vi "TX-ADAR-DETECT.vi"(0 "COMPORT":refnum<visa-resource-name>="COM4", 11 "error in (no error)":errorcluster, 12 "Ant_Sel":i32=1, 13 "Open/Close Serial":bool) -> (3 "string":string="wr txm 0x4A 0x76;wr txm 0x49 0x72", 4 "comport":refnum<visa-resource-name>="COM4", 8 "adc read":dbl=86.0, 15 "error out":errorcluster)   [LabVIEW 2018]
panel:
  out "number":i32=86
  out "after substring":string="56\r\n>\r\n"
  out "All Success":bool=TRUE
  out "output 2":string="\rwr txm 0x4A 0x76\r\n>\rwr txm 0x49 0x72\r\n>\r\rwr txm 0x4A 0x76\r\n>\rwr txm 0x49 0x72\r\n>\rrd txm 0x4B\r\n0x04B: 0x56\r\n>"
  out "Success":bool[](array[boolean])=[TRUE, TRUE, TRUE, TRUE, TRUE, TRUE]
  # "0 for temperature, 13 for Testport"
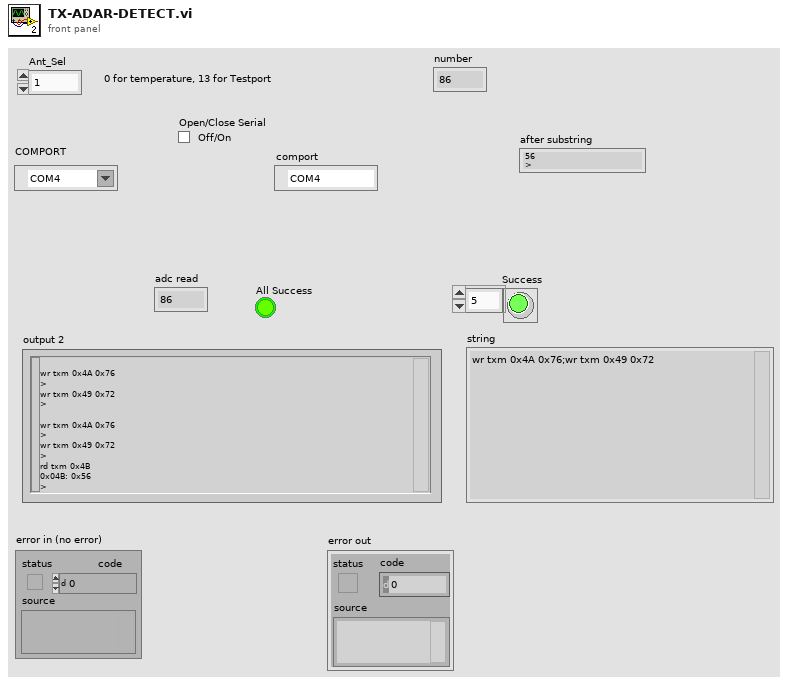
[diagram p1: front panel]
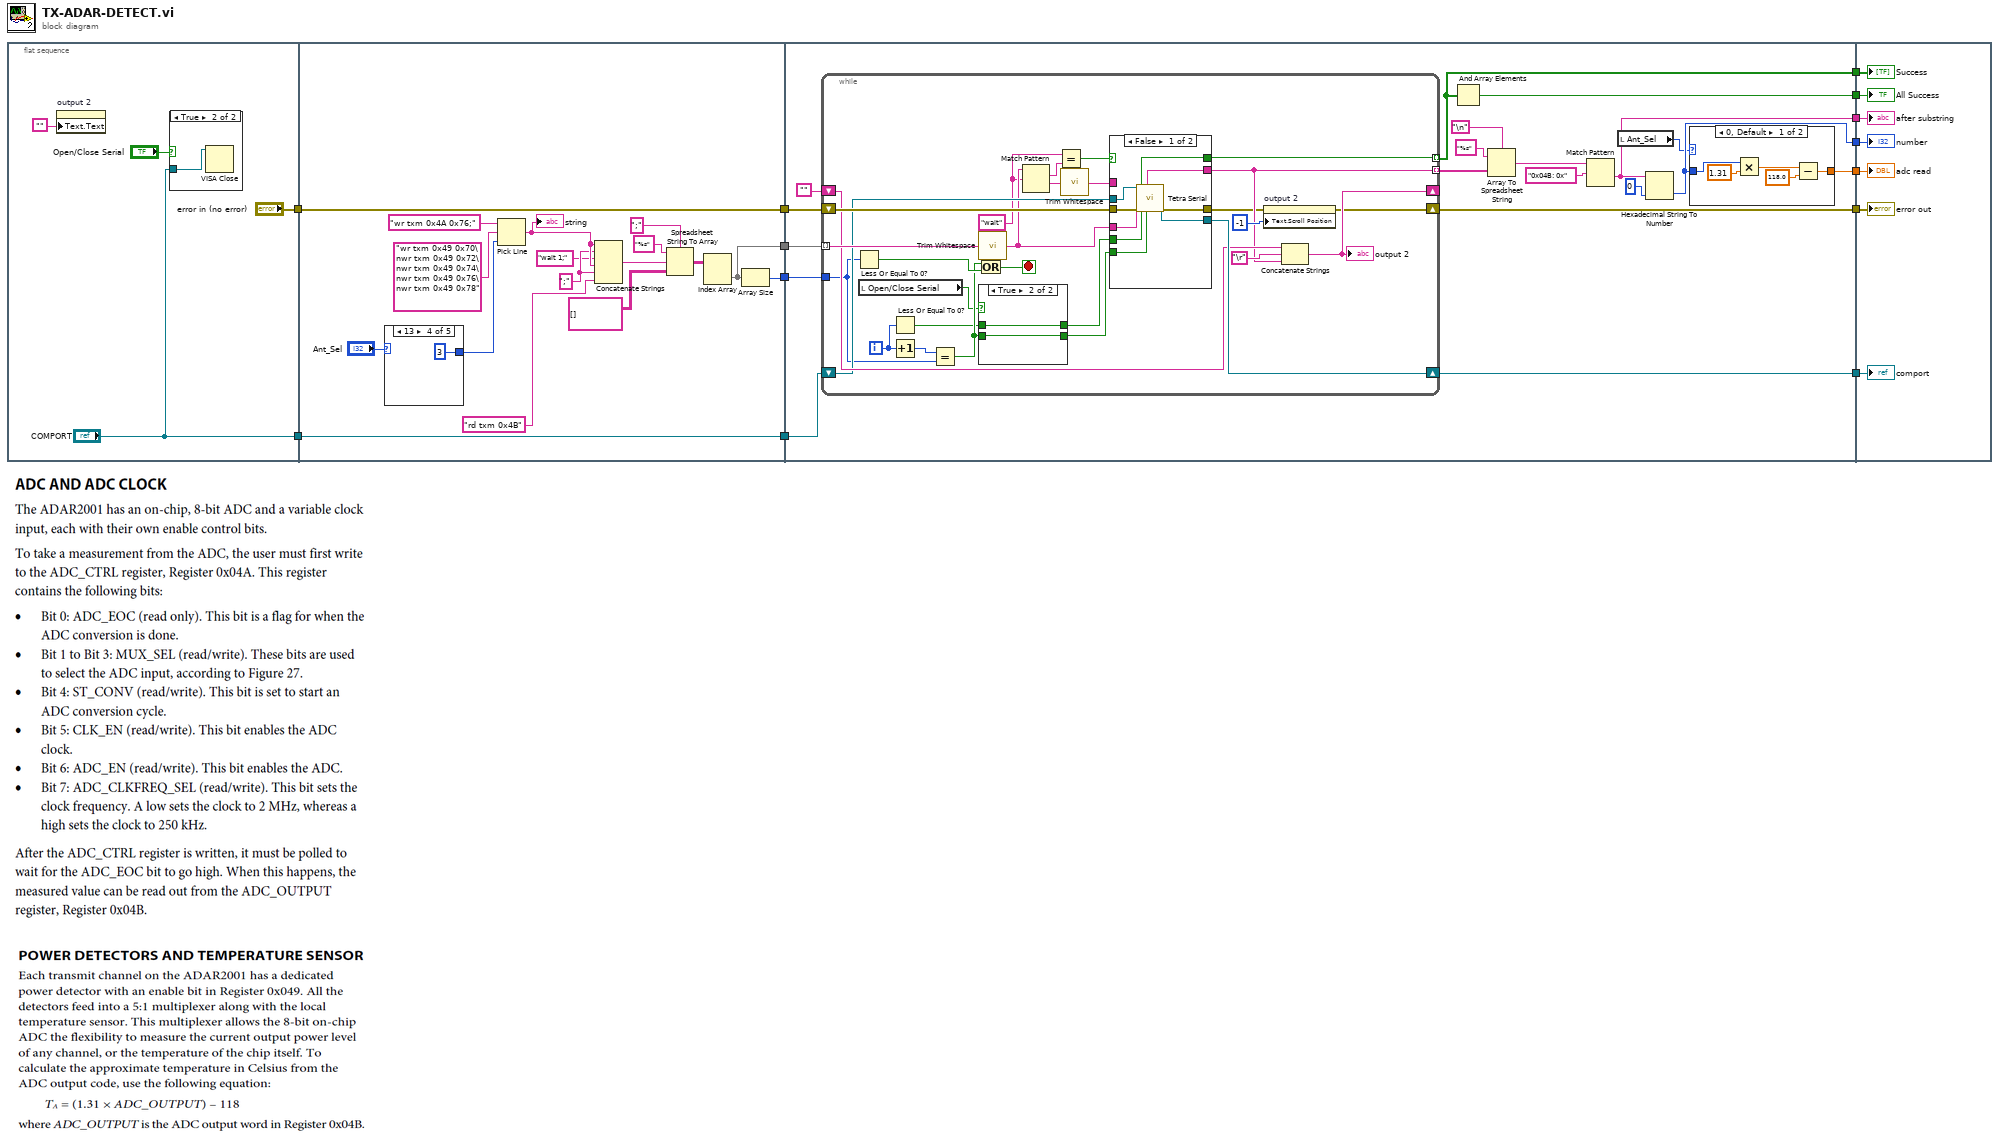
[diagram p0: block diagram]
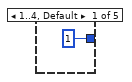
[diagram p3: hidden frame]
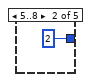
[diagram p4: hidden frame]
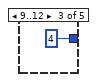
[diagram p5: hidden frame]
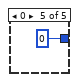
[diagram p6: hidden frame]
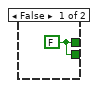
[diagram p8: hidden frame]
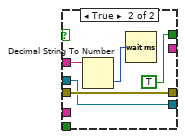
[diagram p9: hidden frame]
diagram:
  n1 = flat-sequence {
    tunnel: ["COMPORT"] -> w2
    tunnel: ["error in (no error)"] -> w1
    tunnel: [w19] -> w6
    tunnel: [w21] -> w5
    tunnel: [w22] -> w4
    tunnel: [w20] -> w3
    tunnel: w2 -> [w20]
    tunnel: w1 -> [w19]
    tunnel: [w59] -> w13
    tunnel: [w57] -> w12
    tunnel: [w52] -> w11
    tunnel: [w51] -> w10
    tunnel: [w46] -> w9
    tunnel: [w44] -> w8
    tunnel: [w43] -> w7
    tunnel: w6 -> [w58]
    tunnel: w5 -> [w56]
    tunnel: w4 -> [w49]
    tunnel: w3 -> [w41]
    tunnel: w13 -> [w111]
    tunnel: w12 -> [w112]
    tunnel: w11 -> [w113]
    tunnel: w10 -> [w114]
    tunnel: w9 -> [w115]
    tunnel: w8 -> [w117]
    tunnel: w7 -> [w116]
    frame #0 {
      n2 = property on="output 2" class="Str"("Text.Text"="") -> ()  [unwired: 2 in, 2 out]
      n3 = case shown="True" "Open/Close Serial" {
        tunnel: "COMPORT" -> [_ w18]
        frame False {
        }
        frame True {
          n4 = VISA Close(VISA resource name=w18) -> ()  [unwired: 1 in, 1 out]
        }
      }
    }
    frame #1 {
      w28 = ";" ("string")
      n5 = case shown="13" "Ant_Sel" {
        tunnel: [1 2 4 3 0] -> w34
        frame 1..4, Default {
        }
        frame 5..8 {
        }
        frame 9..12 {
        }
        frame 13 {
        }
        frame 0 {
        }
      }
      n6 = Pick Line(string ("")="wr txm 0x4A 0x76;" ("Command ( ; seperation)"), multi-line string="wr txm 0x49 0x70\nwr txm 0x49 0x72\nwr txm 0x49 0x74\nwr txm 0x49 0x76\nwr txm 0x49 0x78", line index=w34) -> (output string=w35:string)
      "string" <- w35
      n7 = Concatenate Strings(w35, w28, "wait 1;" ("string"), w35, w28, "rd txm 0x4B" ("string")) -> (w32:string)
      n8 = Spreadsheet String To Array(delimiter (Tab)=";", format string="%s", spreadsheet string=w32, array type (2D Dbl)=string[][] []) -> (array=w31:string[][])
      n9 = Index Array(array=w31) -> (element=w21:string[])  [unwired: 2 in]
      n10 = Array Size(array=w21) -> (size(s)=w22:i32)
    }
    frame #2 {
      n11 = while {
        shift-right: [w71] -> w59
        shift-left: w58 -> [w93]
        shift-right: [w92] -> w57
        shift-left: w41 -> [w82]
        tunnel: [w87] -> w50 mode=indexing
        tunnel: w56 -> [w91] mode=indexing
        tunnel: w49 -> [w80]
        shift-right: [w85] -> _
        shift-left: "" -> [w88]
        tunnel: [w86] -> w52 mode=indexing
        i -> [w83]
        stop <- w81 stop-if-true
        w74 = "wait" ("regular expression")
        n12 = Less Or Equal To 0?(x=w80) -> (x <= 0?=w79:bool)
        n13 = local read "Open/Close Serial"() -> (w66:bool)
        n14 = Less Or Equal To 0?(x=w83) -> (x <= 0?=w67:bool)
        n15 = Increment(x=w83) -> (x+1=w84:i32)
        n16 = Equal?(x=w84, y=w80) -> (x = y?=w70:bool)
        n17 = Or(x=w70, y=w79) -> (x .or. y?=w81:bool)
        n18 = call <vilib>:"Trim Whitespace.vi"("string"=w91) -> ("trimmed string"=w78:string)  [unwired: 1 in]
        n19 = case shown="True" w66 {
          tunnel: w70 -> [_ w96]
          tunnel: [w94 w96] -> w69
          tunnel: [w94 w95] -> w68
          tunnel: w67 -> [_ w95]
          frame False {
            w94 = FALSE
          }
          frame True {
          }
        }
        n20 = Match Pattern(string=w78, regular expression=w74) -> (match substring=w75:string, after substring=w76:string)  [unwired: 1 in, 2 out]
        n21 = Equal?(x=w74, y=w75) -> (x = y?=w77:bool)
        n22 = call <vilib>:"Trim Whitespace.vi"("string"=w76) -> ("trimmed string"=w73:string)  [unwired: 1 in]
        n23 = case shown="False" w77 {
          tunnel: [w105 w108] -> w72
          tunnel: w93 -> [w104 w108]
          tunnel: [w103 w107] -> w92
          tunnel: w68 -> [w102 _]
          tunnel: w69 -> [w101 _]
          tunnel: [w100 _] -> w87
          tunnel: w78 -> [w99 _]
          tunnel: [w98 TRUE ("Success")] -> w86
          tunnel: w82 -> [w97 w107]
          tunnel: w73 -> [_ w110]
          frame False {
            n24 = call "Tetra Serial.vi"("COMPORT"=w97, "error in (no error)"=w104, "Command"=w99, "Open Ser(t)"=w102, "Close Ser(t)"=w101) -> ("Success"=w98:bool, "output"=w100:string, "comport"=w103:refnum<visa-resource-name>, "error out"=w105:errorcluster)  [unwired: 6 in, 1 out]
          }
          frame True {
            n25 = Decimal String To Number(string=w110) -> (number=w109:i32)  [unwired: 2 in, 1 out]
            n26 = Wait (ms)(milliseconds to wait=w109) -> ()  [unwired: 1 out]
          }
        }
        n27 = property on="output 2" class="Str"(error in=w72, "Text.Scroll Position"=-1) -> (error out=w71:errorcluster)  [unwired: 1 in, 1 out]
        n28 = Concatenate Strings(w88, "\r", w87) -> (w85:string)
        "output 2" <- w85
      }
      n29 = And Array Elements(Boolean array=w52) -> (logical AND=w51:bool)
      n30 = Array To Spreadsheet String(delimiter (Tab)="\n", array=w50, 3:"%s" ("format string")) -> (spreadsheet string=w48:string)
      n31 = Match Pattern(string=w48, regular expression="0x04B: 0x") -> (after substring=w46:string)  [unwired: 1 in, 3 out]
      n32 = local read "Ant_Sel"() -> (w42:i32)
      n33 = Hexadecimal String To Number(string=w46, default (0uL)=0 ("default (0 U32)")) -> (number=w44:i32)  [unwired: 1 in, 1 out]
      n34 = case shown="0, Default" w42 {
        tunnel: w44 -> [w64 w65]
        tunnel: [w60 w65] -> w43
        frame 0, Default {
          n35 = Multiply(x=w64, y=1.31) -> (x*y=w62:dbl)
          n36 = Subtract(x=w62, y=118.0) -> (x-y=w60:dbl)
        }
        frame 1..4 {
        }
      }
    }
    frame #3 {
      "error out" <- w111
      "comport" <- w112
      "Success" <- w113
      "All Success" <- w114
      "after substring" <- w115
      "adc read" <- w116
      "number" <- w117
    }
  }
